vi "MB Ethernet Slave Communication.vi"(8 "error in (no error)":errorcluster, 10 "Timeout":i32=5000, 11 "Connection ID":refnum<k5>) -> (0 "error out":errorcluster, 3 "Connection ID (dup)":refnum<k5>)   [LabVIEW 2020]
panel:
  # "VI Name: MB Ethernet Slave Communication.vi\nPurpose: Modbus Ethernet Slave Read.\nReentrant, so we can serve multiple queries in parallel."
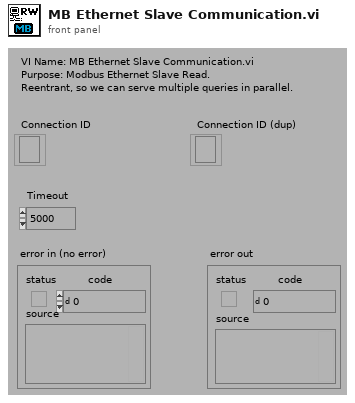
[diagram p1: front panel]
types:
  T1 = typedef "MB Modbus Data Unit.ctl" = cluster{"Function Code":u8, "Data":u8[]}
  T2 = cluster{"Transaction ID":u16, "Protocol ID":u16, "Length":u16, "Unit ID":u8}
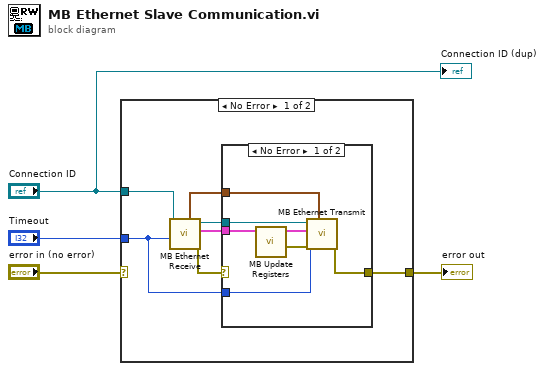
[diagram p0: block diagram]
diagram:
  n1 = case shown="No Error" "error in (no error)" {
    selector: "error in (no error)" -> [_ w20]
    tunnel: "Connection ID" -> [w8 _]
    tunnel: [w11 w20] -> w4
    tunnel: "Timeout" -> [w5 _]
    frame No Error {
      n2 = call "MB Ethernet Receive.vi"("Timeout"=w5, "Connection ID"=w8) -> ("error out"=w7:errorcluster, "Modbus Data Unit"=w9:T1, "Connection ID (dup)"=w10:refnum<k5>, "MBAP Header"=w6:T2)  [unwired: 2 in, 4 out]
      n3 = case shown="No Error" w7 {
        selector: w7 -> [_ w19]
        tunnel: [w18 w19] -> w11
        tunnel: w10 -> [w13 _]
        tunnel: w9 -> [w16 _]
        tunnel: w6 -> [w14 _]
        tunnel: w5 -> [w12 _]
        frame No Error {
          n4 = call "MB Update Registers.vi"("Modbus Data Unit In"=w16) -> ("error out"=w17:errorcluster, "Modbus Data Unit Out"=w15:T1)  [unwired: 1 in, 8 out]
          n5 = call "MB Ethernet Transmit.vi"("MBAP Header"=w14, "error in (no error)"=w17, "Timeout"=w12, "Modbus Data Unit"=w15, "TCP Connection Refnum in"=w13) -> ("error out"=w18:errorcluster)  [unwired: 6 out]
        }
        frame Error {
        }
      }
    }
    frame Error {
    }
  }
  "error out" <- w4
  "Connection ID (dup)" <- "Connection ID"
